vi "subXMLGetSourceDistributionSourceFiles.vi"(9 "Source dist in":map{string, set{string}}(c390), 10 "Build spec name":string, 11 "Refnum in":refnum<k20>) -> (1 "Source dist":map{string, set{string}}(c390))   [LabVIEW 2020, in "SolutionBuilder.lvlib" / "SolutionBuilder.lvclass"]
uses:
  <vilib>/Utility/miscctls.llb/LVMapReplaceAction.ctl
  SolutionBuilder.lvclass
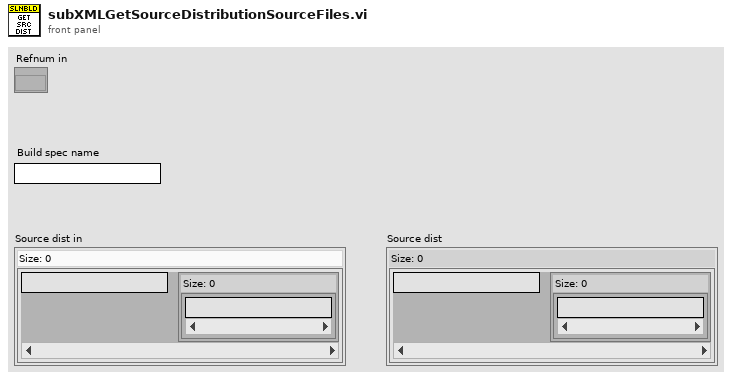
[diagram p1: front panel]
types:
  T1 = typedef "LVMapReplaceAction.ctl" = enum32{"Modify Entry only if found", "Add or Modify Entry", "Delete Entry"}
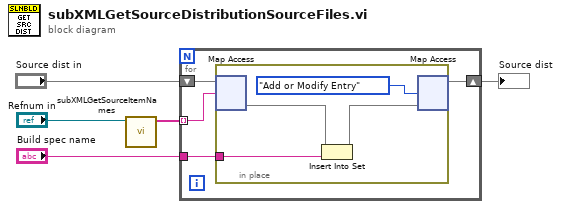
[diagram p0: block diagram]
diagram:
  n1 = call "subXMLGetSourceItemNames.vi"("Refnum in"="Refnum in") -> ("Names"=w5:string[])  [unwired: 10 in]
  n2 = for {
    tunnel: w5 -> [w9] mode=indexing
    tunnel: "Build spec name" -> [w8]
    shift-right: [w6] -> w1
    shift-left: "Source dist in" -> [w7]
    n3 = in-place {
      in-place-border: w8 -> [w12]
      n4 = in-place-map #1(w7, w9) -> (w11:set{string})  [unwired: 1 in, 1 out]
      n5 = Insert Into Set(10:w12, 11:w11) -> (3:w10:set{string})  [unwired: 1 out]
      n6 = in-place-map #1(w10, LVMapReplaceAction."Add or Modify Entry" ("action")) -> (w6:map{string, set{string}})  [unwired: 2 out]
    }
  }
  "Source dist" <- w1
